vi "open_new_h5_file.vi"(8 "error in (no error)":errorcluster, 11 "path":path=path "C:/Documents and Settings/sternovsky/Desktop/New_Data_File.hdf5") -> (0 "error out":errorcluster, 3 "ref":i32)   [LabVIEW 2012]
uses:
  <vilib>/addons/h5labview/H5F_mode.ctl
  <vilib>/addons/h5labview/H5File.lvlib
  <vilib>/addons/h5labview/H5Attrib.lvlib
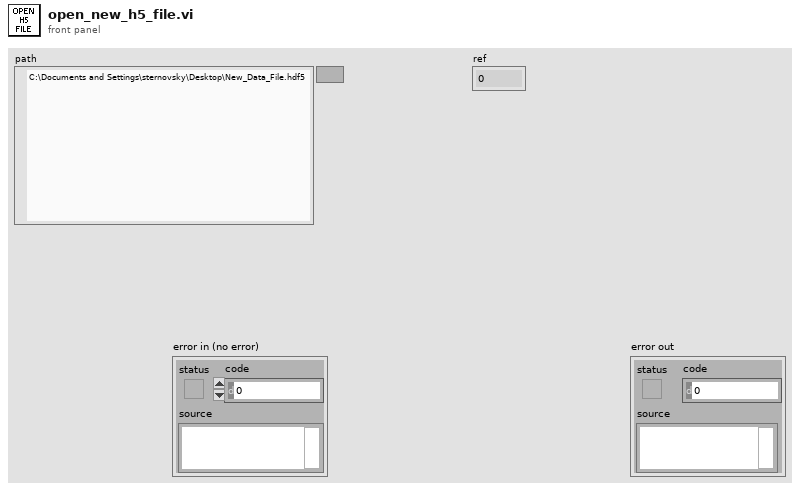
[diagram p1: front panel]
types:
  T1 = typedef "H5File.lvlib/H5F_mode.ctl" = enum16{"read-only", "read-write", "overwrite", "create new", "open or create"}
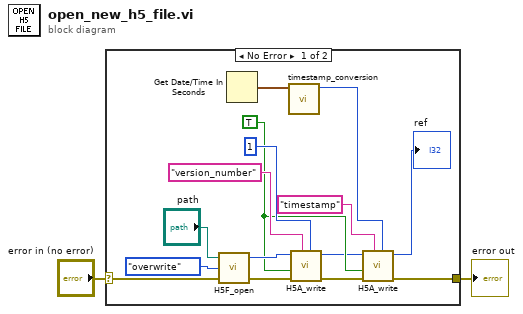
[diagram p0: block diagram]
diagram:
  n1 = case shown="No Error" "error in (no error)" {
    selector: "error in (no error)" -> [w17 w18]
    tunnel: [w9 w18] -> w1
    frame No Error {
      w5 = TRUE ("overwrite? (F)")
      n2 = call <vilib>:"H5F_open.vi"("error in (no error)"=w17, "mode"=H5F_mode."overwrite", "path"="path") -> ("error out"=w11:errorcluster, "ref"=w14:i32)  [unwired: 1 in]
      n3 = Get Date/Time In Seconds() -> (seconds since 1Jan1904=w8:timestamp)
      n4 = call "timestamp_conversion.vi"("Time Stamp"=w8) -> ("Integer Time"=w7:i64)  [unwired: 8 in, 1 out]
      n5 = call <vilib>:"H5A_write.vi"("value"=1, "attrib_name"="version_number", "error in (no error)"=w11, "overwrite? (F)"=w5, "ref"=w14) -> ("error out"=w10:errorcluster, "ref out"=w4:i32)  [unwired: 3 in]
      n6 = call <vilib>:"H5A_write.vi"("value"=w7, "attrib_name"="timestamp", "error in (no error)"=w10, "overwrite? (F)"=w5, "ref"=w4) -> ("error out"=w9:errorcluster, "ref out"=→"ref":i32)  [unwired: 3 in]
    }
    frame Error {
    }
  }
  "error out" <- w1
